vi "EEI EXP5.vi"() -> ()   [LabVIEW 2020]
panel:
  in  "String":string
  out "Output":dbl
  in  "input 1":dbl
  in  "input 2":dbl
  out "current time":timestamp
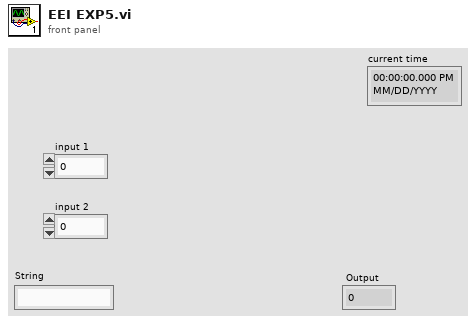
[diagram p1: front panel]
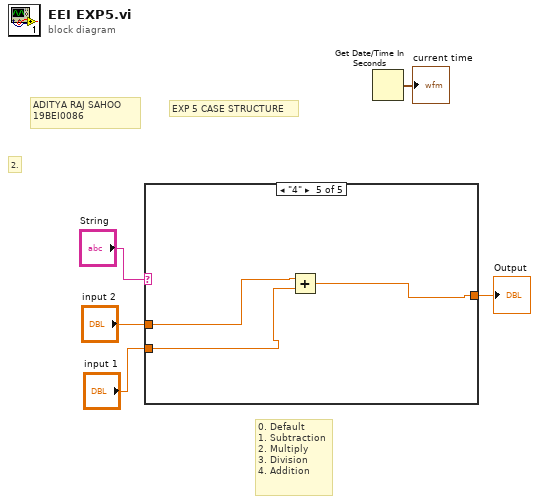
[diagram p0: block diagram]
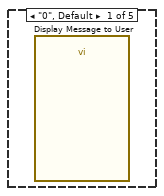
[diagram p2: hidden frame]
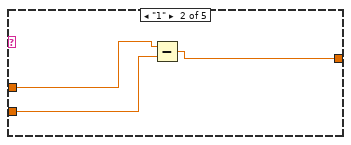
[diagram p3: hidden frame]
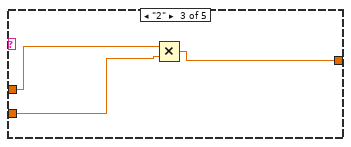
[diagram p4: hidden frame]
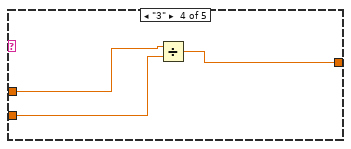
[diagram p5: hidden frame]
diagram:
  # "0. Default\n1. Subtraction\n2. Multiply\n3. Division\n4. Addition"
  # "2."
  # "EXP 5 CASE STRUCTURE"
  # "ADITYA RAJ SAHOO\n19BEI0086"
  n1 = case shown="\"4\"" "String" {
    tunnel: "input 2" -> [_ w8 w11 w14 w17]
    tunnel: "input 1" -> [_ w7 w10 w13 w16]
    tunnel: [_ w6 w9 w12 w15] -> w2
    frame "0", Default {
      n2 = call "Display Message to User"() -> ()  [unwired: 10 in, 2 out]
    }
    frame "1" {
      n3 = Subtract(x=w8, y=w7) -> (x-y=w6:dbl)
    }
    frame "2" {
      n4 = Multiply(x=w11, y=w10) -> (x*y=w9:dbl)
    }
    frame "3" {
      n5 = Divide(x=w14, y=w13) -> (x/y=w12:dbl)
    }
    frame "4" {
      n6 = Add(x=w17, y=w16) -> (x+y=w15:dbl)
    }
  }
  "Output" <- w2
  n7 = Get Date/Time In Seconds() -> (seconds since 1Jan1904=→"current time":timestamp)
